vi "SR830 query reference mode.vi"(8 "error in (no error)":errorcluster, 11 "VISA resource name":refnum<visa-resource-name>) -> (0 "error out":errorcluster, 2 "reference mode":enum16{"external", "internal"}(ring), 3 "VISA resource name out":refnum<visa-resource-name>)   [LabVIEW 2009, in "Lockin SR830.lvclass"]
doc: "Reads the current reference mode (internal or external) of the lock-in amplifier."
uses:
  Lockin SR830.lvclass
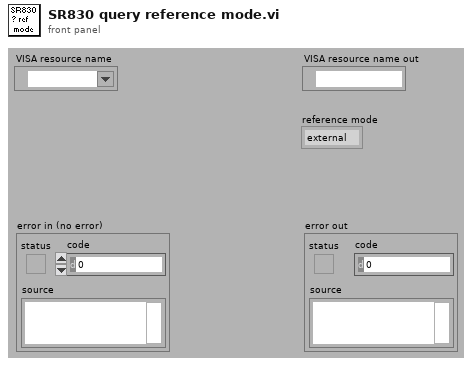
[diagram p1: front panel]
types:
  T1 = typedef "Semaphore RefNum" = refnum<k1>
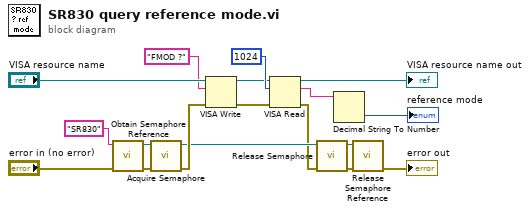
[diagram p0: block diagram]
diagram:
  n1 = call <vilib>:"Obtain Semaphore Reference.vi"("error in (no error)"="error in (no error)", "name (unnamed)"="SR830") -> ("error out"=w12:errorcluster, "semaphore"=w11:T1)  [unwired: 1 in, 3 out]
  n2 = call <vilib>:"Acquire Semaphore.vi"("error in (no error)"=w12, "semaphore"=w11) -> ("error out"=w8:errorcluster, "semaphore out"=w5:T1)  [unwired: 1 in, 3 out]
  n3 = VISA Write(VISA resource name="VISA resource name", write buffer="FMOD ?", error in (no error)=w8) -> (VISA resource name out=w17:refnum<visa-resource-name>, error out=w16:errorcluster)  [unwired: 1 out]
  n4 = VISA Read(VISA resource name=w17, byte count=u32 1024 ("bytes to read (1000)"), error in (no error)=w16) -> (VISA resource name out=→"VISA resource name out":refnum<visa-resource-name>, read buffer=w2:string, error out=w4:errorcluster)  [unwired: 1 out]
  n5 = call <vilib>:"Release Semaphore.vi"("error in (no error)"=w4, "semaphore"=w5) -> ("error out"=w7:errorcluster, "semaphore out"=w6:T1)  [unwired: 4 out]
  n6 = Decimal String To Number(string=w2) -> (number=→"reference mode":i32)  [unwired: 3 out]
  n7 = call <vilib>:"Release Semaphore Reference.vi"("error in (no error)"=w7, "semaphore"=w6) -> ("error out"=→"error out":errorcluster)  [unwired: 9 out]
